vi "AddFailureReference.vi"(8 "error in (no error)":errorcluster, 10 "Id":string, 11 "Measure in":refnum<class "Measure.lvclass">) -> (0 "error out":errorcluster, 2 "FailureReference":refnum<class "FailureReference.lvclass">, 3 "Measure out":refnum<class "Measure.lvclass">)   [LabVIEW 2021, in "ProligentXMLGenerator.lvlib" / "Measure.lvclass"]
uses:
  Measure.lvclass
  Measure.lvclass/Measure.ctl
  Failure/FailureReference/FailureReference.lvclass
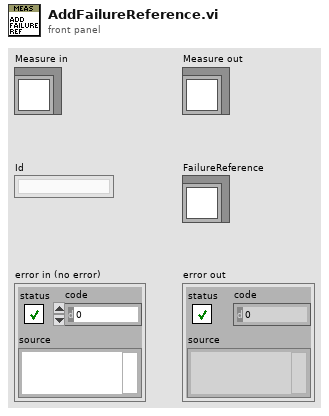
[diagram p1: front panel]
types:
  T1 = typedef "ProligentXMLGenerator.lvlib/Measure.lvclass/Data.ctl" = cluster{"Name":string, "Type":refnum<class "MeasureKind.lvclass">, "Precision":refnum<class "UnsignedByte.lvclass">, "Limit":refnum<class "MeasureLimit.lvclass">, "Characteristics":refnum<class "Characteristic.lvclass">[], "FailureReferences":refnum<class "FailureReference.lvclass">[], "CustomData":refnum<class "CustomData.lvclass">, "MeasureId":refnum<class "Guid.lvclass">, "MeasureTime":refnum<class "DateTime.lvclass">, "Comments":refnum<class "NonNullableString_TruncateAt_255.lvclass">, "Unit":refnum<class "NonEmptyString_30.lvclass">, "Symbol":refnum<class "NonEmptyString_20.lvclass">, "MeasureExecutionStatus":refnum<class "ExecutionStatus.lvclass">}
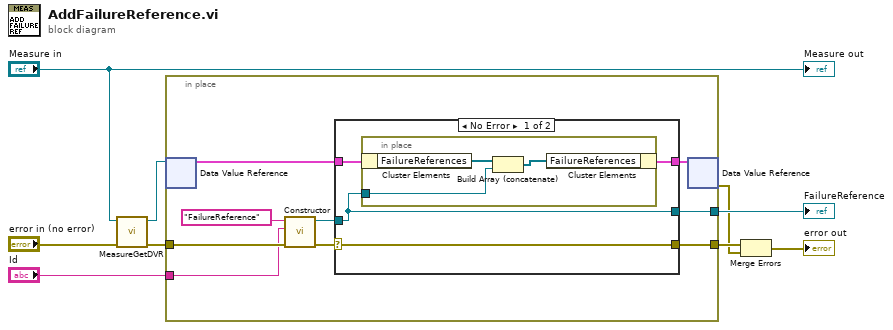
[diagram p0: block diagram]
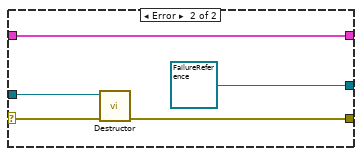
[diagram p2: hidden frame]
diagram:
  n1 = call "MeasureGetDVR.vi"("error in"="error in (no error)", "Measure"="Measure in") -> ("error out"=w7:errorcluster, "DVRReference"=w6:refnum<data-value>)  [unwired: 8 in]
  n2 = in-place "In Place Element Structure" {
    in-place-border: [w18] -> w8
    in-place-border: w7 -> [w11]
    in-place-border: [w15] -> w9
    in-place-border: "Id" -> [w10]
    n3 = in-place-dvr #1(w6) -> (w17:T1)  [unwired: 1 out]
    n4 = call "Constructor.vi"("error in"=w11, "Id"=w10, "Name"="FailureReference") -> ("error out"=w13:errorcluster, "FailureReference out"=w14:refnum<class "FailureReference.lvclass">)  [unwired: 7 in]
    n5 = case shown="No Error" w13 {
      selector: w13 -> [w22 w29]
      tunnel: [w19 w30] -> w16
      tunnel: [w22 w28] -> w18
      tunnel: w14 -> [w21 w27]
      tunnel: w17 -> [w20 w30]
      tunnel: [w21 refnum<class "FailureReference.lvclass"> refnum ("ProligentResultProcessor:FailureReference")] -> w15
      frame No Error {
        n6 = in-place "In Place Element Structure" {
          in-place-border: w21 -> [w25]
          n7 = in-place-cluster #2(w20) -> ("FailureReferences"=w24:refnum<class "FailureReference.lvclass">[])
          n8 = Build Array (concatenate)(w24, w25) -> (w23:refnum<class "FailureReference.lvclass">[])
          n9 = in-place-cluster #2("FailureReferences"=w23) -> (w19:T1)
        }
      }
      frame Error {
        n10 = call "Destructor.vi"("error in"=w29, "FailureReference in"=w27) -> ("error out"=w28:errorcluster)  [unwired: 9 in]
      }
    }
    n11 = in-place-dvr #1(w16) -> (w5:errorcluster)  [unwired: 1 out]
  }
  "FailureReference" <- w9
  n12 = Merge Errors(w8, w5) -> (→"error out":errorcluster)
  "Measure out" <- "Measure in"
